vi "140画曲线.vi"(11 "文件（使用对话框）":path) -> (3 "压机旋铆位移压力图":cluster{dbl[], dbl[]}(graph))   [LabVIEW 2017]
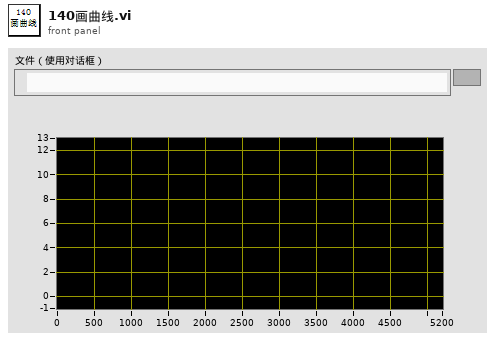
[diagram p1: front panel]
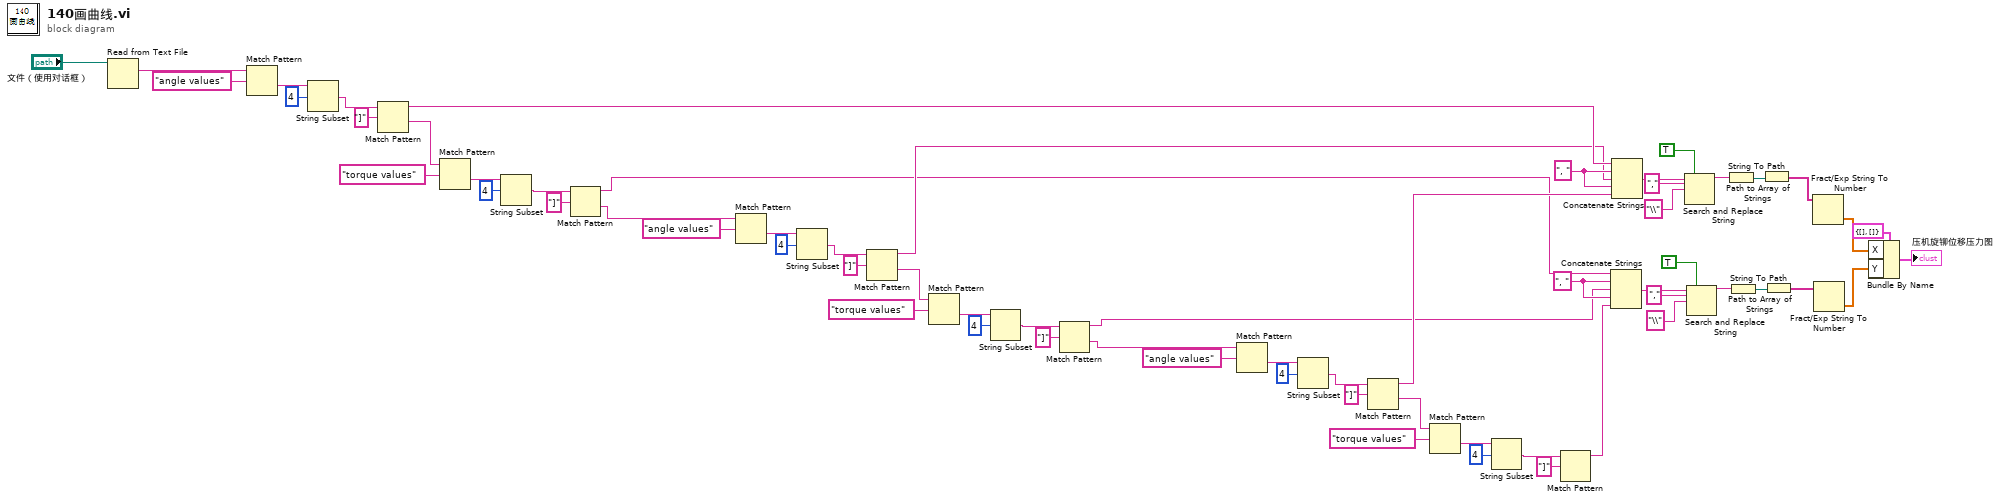
[diagram p0: block diagram]
diagram:
  w25 = ", " ("字符串")
  w26 = ", " ("字符串")
  n1 = Read from Text File(file (use dialog)="文件（使用对话框）") -> (text=w62:string)  [unwired: 3 in, 3 out]
  n2 = Match Pattern(string=w62, regular expression="angle values" ("正则表达式")) -> (after substring=w60:string)  [unwired: 1 in, 3 out]
  n3 = String Subset(string=w60, offset (0)=4 ("偏移量(0)")) -> (substring=w58:string)  [unwired: 1 in]
  n4 = Match Pattern(string=w58, regular expression="]" ("正则表达式")) -> (before substring=w24:string, after substring=w53:string)  [unwired: 1 in, 2 out]
  n5 = Match Pattern(string=w53, regular expression="torque values" ("正则表达式")) -> (after substring=w55:string)  [unwired: 1 in, 3 out]
  n6 = String Subset(string=w55, offset (0)=4 ("偏移量(0)")) -> (substring=w51:string)  [unwired: 1 in]
  n7 = Match Pattern(string=w51, regular expression="]" ("正则表达式")) -> (before substring=w21:string, after substring=w45:string)  [unwired: 1 in, 2 out]
  n8 = Match Pattern(string=w45, regular expression="angle values" ("正则表达式")) -> (after substring=w47:string)  [unwired: 1 in, 3 out]
  n9 = String Subset(string=w47, offset (0)=4 ("偏移量(0)")) -> (substring=w49:string)  [unwired: 1 in]
  n10 = Match Pattern(string=w49, regular expression="]" ("正则表达式")) -> (before substring=w23:string, after substring=w39:string)  [unwired: 1 in, 2 out]
  n11 = Match Pattern(string=w39, regular expression="torque values" ("正则表达式")) -> (after substring=w41:string)  [unwired: 1 in, 3 out]
  n12 = String Subset(string=w41, offset (0)=4 ("偏移量(0)")) -> (substring=w44:string)  [unwired: 1 in]
  n13 = Match Pattern(string=w44, regular expression="]" ("正则表达式")) -> (before substring=w20:string, after substring=w27:string)  [unwired: 1 in, 2 out]
  n14 = Match Pattern(string=w27, regular expression="angle values" ("正则表达式")) -> (after substring=w31:string)  [unwired: 1 in, 3 out]
  n15 = String Subset(string=w31, offset (0)=4 ("偏移量(0)")) -> (substring=w29:string)  [unwired: 1 in]
  n16 = Match Pattern(string=w29, regular expression="]" ("正则表达式")) -> (before substring=w22:string, after substring=w38:string)  [unwired: 1 in, 2 out]
  n17 = Match Pattern(string=w38, regular expression="torque values" ("正则表达式")) -> (after substring=w36:string)  [unwired: 1 in, 3 out]
  n18 = String Subset(string=w36, offset (0)=4 ("偏移量(0)")) -> (substring=w33:string)  [unwired: 1 in]
  n19 = Match Pattern(string=w33, regular expression="]" ("正则表达式")) -> (before substring=w19:string)  [unwired: 1 in, 3 out]
  n20 = Concatenate Strings(w21, w25, w20, w25, w19) -> (w7:string)
  n21 = Concatenate Strings(w24, w26, w23, w26, w22) -> (w18:string)
  n22 = Search and Replace String(replace all?=TRUE ("替换全部？(F)"), input string=w18, search string="," ("搜索字符串"), replace string="\\" ("替换字符串(\"\")")) -> (result string=w15:string)  [unwired: 4 in, 3 out]
  n23 = Search and Replace String(replace all?=TRUE ("替换全部？(F)"), input string=w7, search string="," ("搜索字符串"), replace string="\\" ("替换字符串(\"\")")) -> (result string=w10:string)  [unwired: 4 in, 3 out]
  n24 = String To Path(string=w15) -> (path=w14:path)
  n25 = String To Path(string=w10) -> (path=w11:path)
  n26 = Path to Array of Strings(0:w14) -> (2:w4:string[])  [unwired: 1 out]
  n27 = Path to Array of Strings(0:w11) -> (2:w2:string[])  [unwired: 1 out]
  n28 = Fract/Exp String To Number(string=w4) -> (number=w3:dbl[])  [unwired: 3 in, 1 out]
  n29 = Fract/Exp String To Number(string=w2) -> (number=w1:dbl[])  [unwired: 3 in, 1 out]
  n30 = Bundle By Name(cluster=cluster{"X":dbl[], "Y":dbl[]} {"X"=[], "Y"=[]}, "X"=w3, "Y"=w1) -> (→"压机旋铆位移压力图":cluster{"X":dbl[], "Y":dbl[]})
